vi "_PC_MS_SubVI exeInit.vi"(7 "Auto Index":refnum<vi>, 8 "error in (no error)":errorcluster, 9 "Ionisation Ref":refnum<vi>, 10 "TIC Ref":refnum<vi>, 11 "Mass Spetrum Ref":refnum<vi>) -> (0 "error out":errorcluster)   [LabVIEW 2018]
uses:
  PublicSubVI/Class/FileManager/FM/ctl/_PC_Pub_FM ctrlFileRefnumEnum.ctl
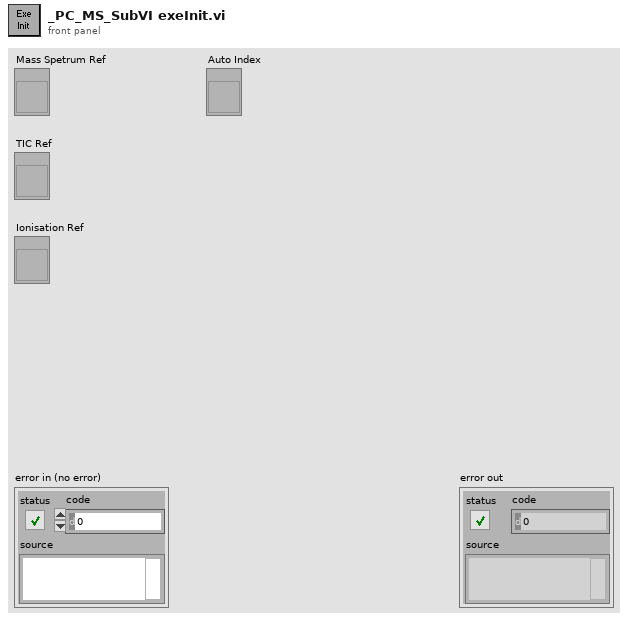
[diagram p1: front panel]
types:
  T1 = typedef "_PC_Pub_FM ctrlFileRefnumEnum.ctl" = enum16{"init", "checkFileName", "updFileName", "updWorkFolder", "updDataItems", "addNewFileName", "addSerialNum"}
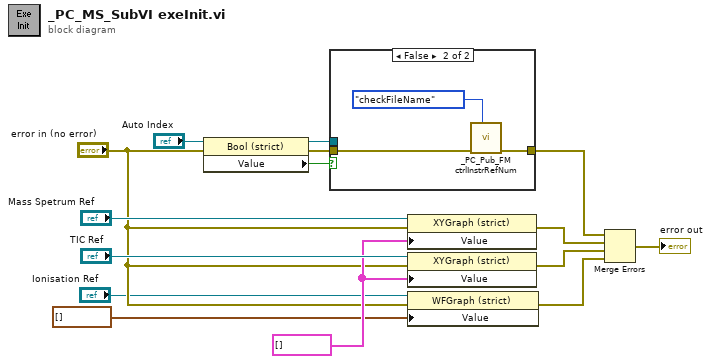
[diagram p0: block diagram]
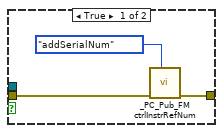
[diagram p2: hidden frame]
diagram:
  w9 = cluster{"X":dbl[], "Y":dbl[]}[] [] ("Value")
  n1 = property class="Bool (strict)"(reference="Auto Index", error in="error in (no error)") -> (reference out=w5:refnum<vi>, error out=w4:errorcluster, "Value"=w6:bool)
  n2 = case shown="False" w6 {
    tunnel: w5 -> [_ _]
    tunnel: w4 -> [w18 w21]
    tunnel: [w17 w20] -> w1
    frame True {
      n3 = call "_PC_Pub_FM ctrlInstrRefNum.vi"("function"=_PC_Pub_FM_ctrlFileRefnumEnum."addSerialNum", "error in (no error)"=w18) -> ("error out"=w17:errorcluster)  [unwired: 9 in]
    }
    frame False {
      n4 = call "_PC_Pub_FM ctrlInstrRefNum.vi"("function"=_PC_Pub_FM_ctrlFileRefnumEnum."checkFileName", "error in (no error)"=w21) -> ("error out"=w20:errorcluster)  [unwired: 9 in]
    }
  }
  n5 = property class="XYGraph (strict)"(reference="Mass Spetrum Ref", error in="error in (no error)", "Value"=w9) -> (error out=w13:errorcluster)  [unwired: 1 out]
  n6 = property class="XYGraph (strict)"(reference="TIC Ref", error in="error in (no error)", "Value"=w9) -> (error out=w14:errorcluster)  [unwired: 1 out]
  n7 = property class="WFGraph (strict)"(reference="Ionisation Ref", error in="error in (no error)", "Value"=waveform(dbl)[] []) -> (error out=w15:errorcluster)  [unwired: 1 out]
  n8 = Merge Errors(w1, w13, w14, w15) -> (→"error out":errorcluster)
